vi "openConnection_Subscriber.vi"(8 "error in (no error)":errorcluster, 10 "TCP address":string="tcp://127.0.0.1:5555", 11 "LabVIEW-Python-Interface in":refnum<class "PyLVi.lvclass">) -> (0 "error out":errorcluster, 2 "connected":bool, 3 "LabVIEW-Python-Interface out":refnum<class "PyLVi.lvclass">)   [LabVIEW 2016, in "PyLVi.lvlib" / "PyLVi.lvclass"]
doc: "\"receive timeout\": timeout in ms. If value is negative, no timeout is set."
uses:
  PyLVi.lvclass
  <vilib>/addons/zeromq/socket_type.ctl
  <vilib>/addons/zeromq/socket_options.ctl
  PyLVi.lvclass/PyLVi.ctl
  <vilib>/addons/zeromq/zmq_context.lvclass
  <vilib>/addons/zeromq/zeromq.lvlib
  <vilib>/addons/zeromq/zmq_socket.lvclass
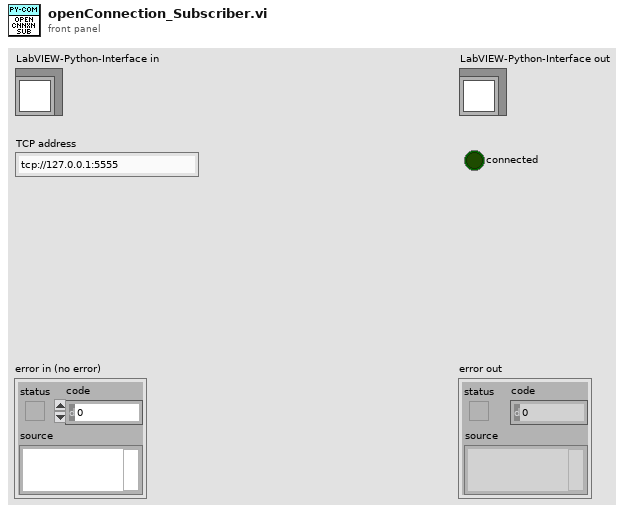
[diagram p1: front panel]
types:
  T1 = typedef "zeromq.lvlib/socket_options.ctl" = enum8{"NONE", "ZMQ_HWM", "<2>", "ZMQ_SWAP", "ZMQ_AFFINITY", "ZMQ_IDENTITY", "ZMQ_SUBSCRIBE", "ZMQ_UNSUBSCRIBE", "ZMQ_RATE", "ZMQ_RECOVERY_IVL", "ZMQ_MCAST_LOOP", "ZMQ_SNDBUF", "ZMQ_RCVBUF", "ZMQ_RCVMORE", "ZMQ_FD", "ZMQ_EVENTS", "ZMQ_TYPE", "ZMQ_LINGER", "ZMQ_RECONNECT_IVL", "ZMQ_BACKLOG", "ZMQ_RECOVERY_IVL_MSEC", "ZMQ_RECONNECT_IVL_MAX", "ZMQ_MAXMSGSIZE", "ZMQ_SNDHWM", "ZMQ_RCVHWM", "ZMQ_MULTICAST_HOPS", "<26>", "ZMQ_RCVTIMEO", "ZMQ_SNDTIMEO", "<29>", "<30>", "ZMQ_IPV4ONLY", "ZMQ_LAST_ENDPOINT", "ZMQ_ROUTER_MANDATORY", "ZMQ_TCP_KEEPALIVE", "ZMQ_TCP_KEEPALIVE_CNT", "ZMQ_TCP_KEEPALIVE_IDLE", "ZMQ_TCP_KEEPALIVE_INTVL", "ZMQ_TCP_ACCEPT_FILTER", "ZMQ_DELAY_ATTACH_ON_CONNECT", "ZMQ_XPUB_VERBOSE"}
  T2 = typedef "zeromq.lvlib/socket_type.ctl" = enum8{"ZMQ_PAIR", "ZMQ_PUB", "ZMQ_SUB", "ZMQ_REQ", "ZMQ_REP", "ZMQ_DEALER", "ZMQ_ROUTER", "ZMQ_PULL", "ZMQ_PUSH", "ZMQ_XPUB", "ZMQ_XSUB"}
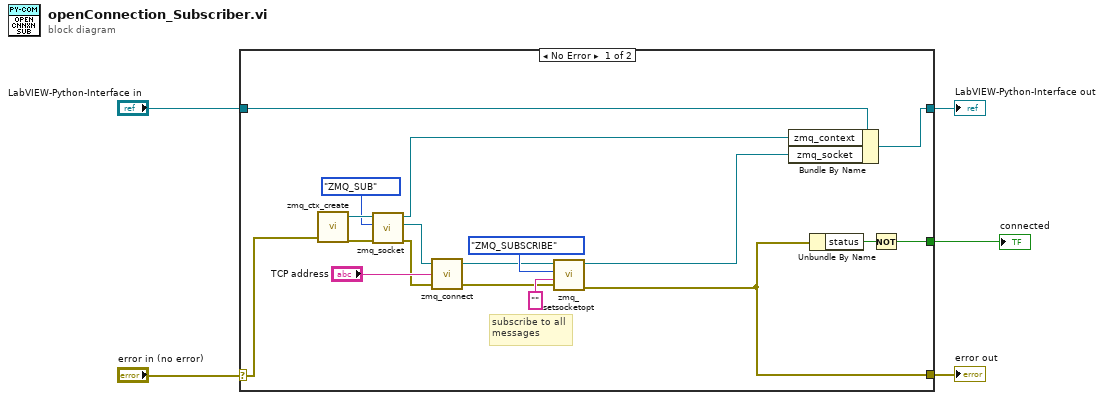
[diagram p0: block diagram]
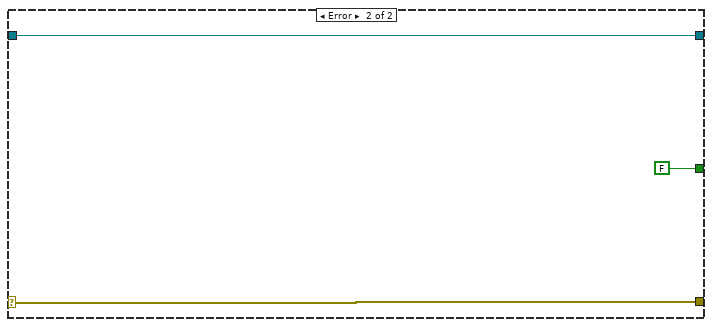
[diagram p2: hidden frame]
diagram:
  n1 = case shown="No Error" "error in (no error)" {
    selector: "error in (no error)" -> [w17 w26]
    tunnel: [w7 w26] -> w4
    tunnel: [w14 w25] -> w2
    tunnel: "LabVIEW-Python-Interface in" -> [w16 w25]
    tunnel: [w12 FALSE ("connected")] -> w1
    frame No Error {
      # "subscribe to all\nmessages"
      n2 = call <vilib>:"zmq_ctx_create.vi"("error in"=w17) -> ("error out"=w22:errorcluster, "context out"=w23:refnum<class "zmq_context.lvclass">)  [unwired: 3 in]
      n3 = call <vilib>:"zmq_socket.vi"("error in"=w22, "socket type"=socket_type."ZMQ_SUB", "context in"=w23) -> ("error out"=w18:errorcluster, "socket out"=w19:refnum<class "zmq_socket.lvclass">, "context out"=w15:refnum<class "zmq_context.lvclass">)  [unwired: 2 in]
      n4 = call <vilib>:"zmq_connect.vi"("error in"=w18, "endpoint"="TCP address", "socket in"=w19) -> ("error out"=w8:errorcluster, "socket out"=w9:refnum<class "zmq_socket.lvclass">)  [unwired: 1 in]
      n5 = call <vilib>:"zmq_setsocketopt.vi"("error in"=w8, "value"="", "option"=socket_options."ZMQ_SUBSCRIBE", "socket in"=w9) -> ("error out"=w7:errorcluster, "socket out"=w6:refnum<class "zmq_socket.lvclass">)  [unwired: 2 in]
      n6 = Bundle By Name(cluster=w16, "zmq_context"=w15, "zmq_socket"=w6) -> (w14:refnum<class "PyLVi.lvclass">)
      n7 = Unbundle By Name(w7) -> ("status"=w13:bool)
      n8 = Not(x=w13) -> (.not. x?=w12:bool)
    }
    frame Error {
    }
  }
  "error out" <- w4
  "LabVIEW-Python-Interface out" <- w2
  "connected" <- w1
